vi "Actor Core.vi"(8 "error in":errorcluster, 11 "IED Test in":refnum<class "IED Test.lvclass">) -> (0 "error out":errorcluster, 3 "Actor out":refnum<class "Actor.lvclass">)   [LabVIEW 2018, in "IED Test Framework.lvlib" / "IED Test.lvclass"]
doc: "(<B>Filename</B>: Actor Framework.lvlib:Actor.lvclass:Actor Core.vi)\n\nReceives messages to the actor, reacts to them, and initiates any error handling that may shut the actor down.\n\nDescendant classes may override this VI to append parallel tasks for the actor to complete while it handles messages. Overrides use the Call Parent Method node."
uses:
  IED Test.lvclass
  C:/Program Files (x86)/National Instruments/LabVIEW 2018/vi.lib/ActorFramework/Actor/Actor.lvclass
  <vilib>/ActorFramework/Actor/Actor.lvclass
  Controls/Tests Cluster.ctl
  IED Test.lvclass/IED Test.ctl
  Controls/Available Tests.ctl
  Controls/Test Result.ctl
  <vilib>/ActorFramework/Actor/Actor.lvclass/Actor.ctl
  <vilib>/ActorFramework/Message Enqueuer/Message Enqueuer.lvclass/Message Enqueuer.ctl
  <vilib>/ActorFramework/Message Enqueuer/Init from Existing Queue.vi
  <vilib>/ActorFramework/Message Enqueuer/Enqueue.vi
  <vilib>/ActorFramework/Stop Msg/Stop Msg.lvclass
  C:/Program Files (x86)/National Instruments/LabVIEW 2018/vi.lib/ActorFramework/Message/Message.lvclass
  <vilib>/ActorFramework/Message Priority Queue/Priority Enqueue.vi
  EMS Generic Actor/EMS Generic/EMS Generic.lvclass
  <vilib>/ActorFramework/Message Enqueuer/Message Enqueuer.lvclass
panel:
  in  "OK Button":bool
  out "Tests":T1
  out "Results":string[][](table)
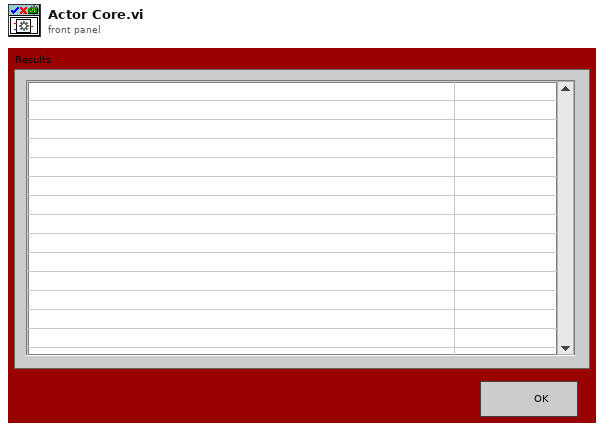
[diagram p1: front panel]
types:
  T1 = typedef "IED Test Framework.lvlib/IED Test.lvclass/Tests Cluster.ctl" = cluster{"Generic IED":bool, "Generic DER":bool, "Energy Storage":bool, "PV":bool, "Generator":bool, "Relay":bool, "Smart Relay":bool, "PCC":bool, "Meter":bool, "Load":bool, "HVAC":bool, "Price Data":bool, "Forecast Data":bool}
  T2 = typedef "IED Test Framework.lvlib/IED Test.lvclass/Available Tests.ctl" = enum16{"Generic IED", "Generic DER", "Energy Storage", "PV", "Generator", "Relay", "Smart Relay", "PCC", "Meter", "Load", "HVAC", "Price Data", "Forecast Data"}
  T3 = typedef "IED Test Framework.lvlib/IED Test.lvclass/Test Result.ctl" = enum16{"Invalid", "Success", "Failure", "Error", "Timeout"}
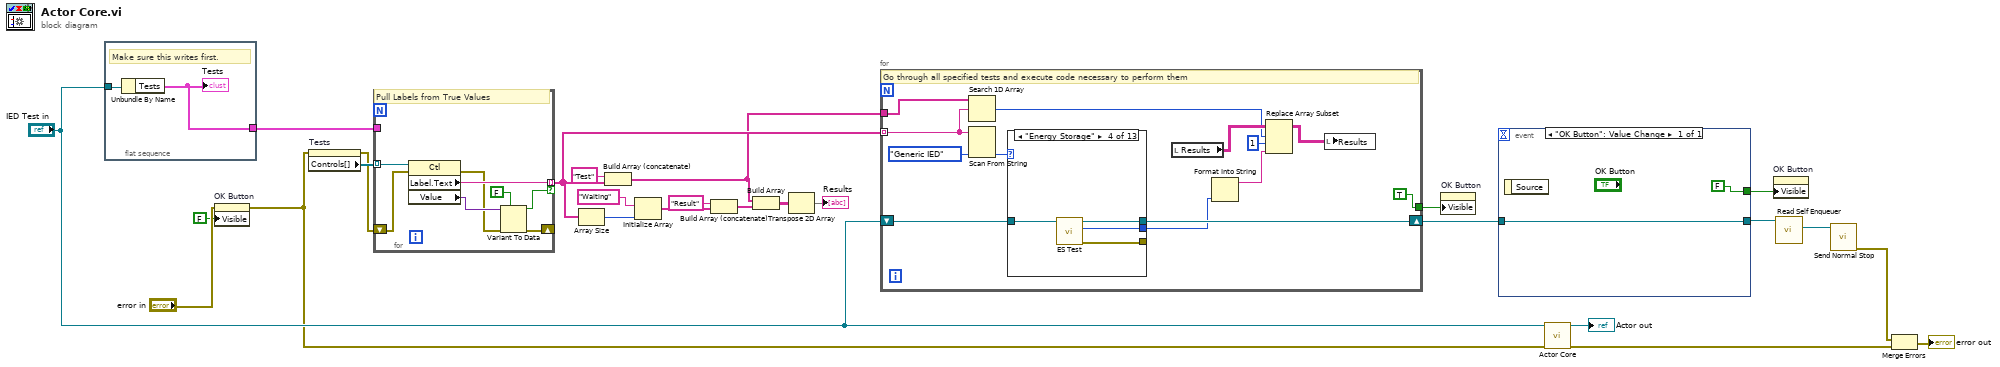
[diagram p0: block diagram]
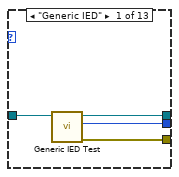
[diagram p2: hidden frame]
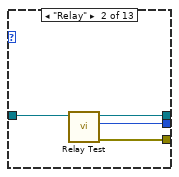
[diagram p3: hidden frame]
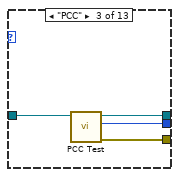
[diagram p4: hidden frame]
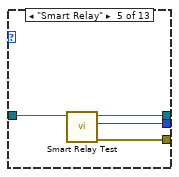
[diagram p5: hidden frame]
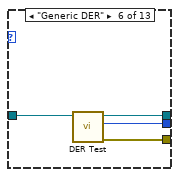
[diagram p6: hidden frame]
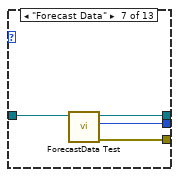
[diagram p7: hidden frame]
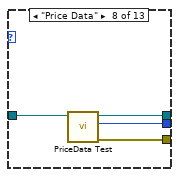
[diagram p8: hidden frame]
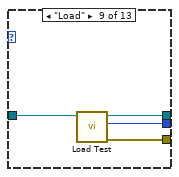
[diagram p9: hidden frame]
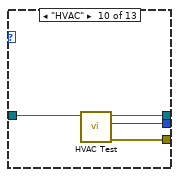
[diagram p10: hidden frame]
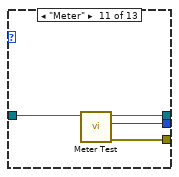
[diagram p11: hidden frame]
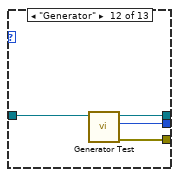
[diagram p12: hidden frame]
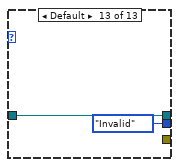
[diagram p13: hidden frame]
diagram:
  n1 = flat-sequence {
    tunnel: "IED Test in" -> [w28]
    tunnel: [w27] -> w14
    frame #0 {
      # "Make sure this writes first."
      n2 = Unbundle By Name(w28) -> ("Tests"=w27:T1)
      "Tests" <- w27
    }
  }
  n3 = property on="OK Button" class="Bool"(error in="error in", "Visible"=FALSE) -> (error out=w9:errorcluster)  [unwired: 1 in, 1 out]
  n4 = property on="Tests" class="Clust (strict)"(error in=w9) -> (error out=w15:errorcluster, "Controls[]"=w24:refnum<vi>[])  [unwired: 1 in, 1 out]
  n5 = for {
    tunnel: w24 -> [w36] mode=indexing
    tunnel: [w33] -> w13 mode=indexing if=w32
    shift-right: [w31] -> _
    shift-left: w15 -> [w30]
    tunnel: w14 -> [_]
    # "Pull Labels from True Values"
    n6 = property class="Ctl"(reference=w36, error in=w30) -> (error out=w29:errorcluster, "Label.Text"=w33:string, "Value"=w34:variant)  [unwired: 1 out]
    n7 = Variant To Data(error in=w29, type=FALSE, Variant=w34) -> (data=w32:bool, error out=w31:errorcluster)
  }
  n8 = Array Size(array=w13) -> (size(s)=w21:i32)
  n9 = Build Array (concatenate)("Test" ("string"), w13) -> (w3:string[])
  n10 = Initialize Array("Waiting" ("string"), w21) -> (w19:string[])
  n11 = Build Array (concatenate)("Result" ("string"), w19) -> (w18:string[])
  n12 = Build Array(w3, w18) -> (w17:string[][])
  n13 = Transpose 2D Array(2D array=w17) -> (transposed array=→"Results":string[][])
  n14 = for {
    tunnel: w13 -> [w44] mode=indexing
    shift-right: [w46] -> w11
    shift-left: "IED Test in" -> [w47]
    tunnel: w3 -> [w45]
    tunnel: [TRUE ("Visible")] -> w2
    # "Go through all specified tests and execute code necessary to perform them"
    n15 = Search 1D Array(1D array=w45, element=w44) -> (index of element=w42:i32)  [unwired: 1 in]
    n16 = Scan From String(input string=w44, default 1=Available_Tests."Generic IED" ("Tests")) -> (output 1=w48:T2)  [unwired: 3 in, 3 out]
    n17 = case shown="\"Energy Storage\"" w48 {
      tunnel: w47 -> [w53 w57 w61 w65 w69 w73 w77 w81 w85 w89 w93 w97 w99]
      tunnel: [w52 w56 w60 w64 w68 w72 w76 w79 w84 w88 w92 w96 w99] -> w46
      tunnel: [w50 w55 w59 w63 w67 w71 w75 w80 w82 w86 w90 w94 _] -> _
      tunnel: [w51 w54 w58 w62 w66 w70 w74 w78 w83 w87 w91 w95 Test_Result."Invalid" ("Test Result")] -> w40
      frame "Generic IED" {
        n18 = call "Generic IED Test.vi"("IED Test in"=w53) -> ("error out"=w50:errorcluster, "Test Result"=w51:T3, "IED Test out"=w52:refnum<class "IED Test.lvclass">)  [unwired: 8 in]
      }
      frame "Relay" {
        n19 = call "Relay Test.vi"("IED Test in"=w57) -> ("error out"=w55:errorcluster, "Test Result"=w54:T3, "IED Test out"=w56:refnum<class "IED Test.lvclass">)  [unwired: 8 in]
      }
      frame "PCC" {
        n20 = call "PCC Test.vi"("IED Test in"=w61) -> ("error out"=w59:errorcluster, "Test Result"=w58:T3, "IED Test out"=w60:refnum<class "IED Test.lvclass">)  [unwired: 8 in]
      }
      frame "Energy Storage" {
        n21 = call "ES Test.vi"("IED Test in"=w65) -> ("error out"=w63:errorcluster, "Test Result"=w62:T3, "IED Test out"=w64:refnum<class "IED Test.lvclass">)  [unwired: 8 in]
      }
      frame "Smart Relay" {
        n22 = call "Smart Relay Test.vi"("IED Test in"=w69) -> ("error out"=w67:errorcluster, "Test Result"=w66:T3, "IED Test out"=w68:refnum<class "IED Test.lvclass">)  [unwired: 8 in]
      }
      frame "Generic DER" {
        n23 = call "DER Test.vi"("IED Test in"=w73) -> ("error out"=w71:errorcluster, "Test Result"=w70:T3, "IED Test out"=w72:refnum<class "IED Test.lvclass">)  [unwired: 8 in]
      }
      frame "Forecast Data" {
        n24 = call "ForecastData Test.vi"("IED Test in"=w77) -> ("error out"=w75:errorcluster, "Test Result"=w74:T3, "IED Test out"=w76:refnum<class "IED Test.lvclass">)  [unwired: 8 in]
      }
      frame "Price Data" {
        n25 = call "PriceData Test.vi"("IED Test in"=w81) -> ("error out"=w80:errorcluster, "Test Result"=w78:T3, "IED Test out"=w79:refnum<class "IED Test.lvclass">)  [unwired: 8 in]
      }
      frame "Load" {
        n26 = call "Load Test.vi"("IED Test in"=w85) -> ("error out"=w82:errorcluster, "Test Result"=w83:T3, "IED Test out"=w84:refnum<class "IED Test.lvclass">)  [unwired: 8 in]
      }
      frame "HVAC" {
        n27 = call "HVAC Test.vi"("IED Test in"=w89) -> ("error out"=w86:errorcluster, "Test Result"=w87:T3, "IED Test out"=w88:refnum<class "IED Test.lvclass">)  [unwired: 8 in]
      }
      frame "Meter" {
        n28 = call "Meter Test.vi"("IED Test in"=w93) -> ("error out"=w90:errorcluster, "Test Result"=w91:T3, "IED Test out"=w92:refnum<class "IED Test.lvclass">)  [unwired: 8 in]
      }
      frame "Generator" {
        n29 = call "Generator Test.vi"("IED Test in"=w97) -> ("error out"=w94:errorcluster, "Test Result"=w95:T3, "IED Test out"=w96:refnum<class "IED Test.lvclass">)  [unwired: 8 in]
      }
      frame Default {
      }
    }
    n30 = local read "Results"() -> (w43:string[][])
    n31 = Format Into String(w40) -> (resulting string=w39:string)  [unwired: 3 in, 1 out]
    n32 = Replace Array Subset(array=w43, new element=w39, index (row)=w42, index (col)=1 ("disabled index (col)")) -> (w38:string[][])
    n33 = local write "Results"(w38) -> ()
  }
  n34 = property on="OK Button" class="Bool"("Visible"=w2) -> ()  [unwired: 2 in, 2 out]
  n35 = event shown="[0] \"OK Button\": Value Change" {
    selector: _ -> [_]
    dyn-events: _ -> [_]
    timeout: _ -> [_]
    tunnel: w11 -> [w101]
    tunnel: [w101] -> w7
    tunnel: [FALSE ("Visible")] -> w1
    event "OK Button": Value Change {
      n36 = event-data() -> ()  [unwired: 1 in, 1 out]
    }
  }
  n37 = call-parent "Actor Core.vi"("error in"=w9, "Actor in"="IED Test in") -> ("error out"=w26:errorcluster, "Actor out"=→"Actor out":refnum<class "Actor.lvclass">)  [unwired: 8 in]
  n38 = property on="OK Button" class="Bool"("Visible"=w1) -> ()  [unwired: 2 in, 2 out]
  n39 = call <vilib>:"Read Self Enqueuer.vi"("Actor"=w7) -> ("Self Enqueuer"=w6:refnum<class "Message Enqueuer.lvclass">)  [unwired: 10 in]
  n40 = call <vilib>:"Send Normal Stop.vi"("Message Enqueuer"=w6) -> ("error out"=w4:errorcluster)  [unwired: 10 in]
  n41 = Merge Errors(w4, w26) -> (→"error out":errorcluster)
